vi "Cocktail.vi"() -> ()   [LabVIEW 2018]
uses:
  pathGlobal.vi
  <vilib>/Utility/config.llb/Read Key (Double).vi
  <vilib>/Utility/config.llb/Write Key (Double).vi
  <vilib>/Utility/config.llb/NI_LVConfig.lvlib
panel:
  in  "Power":bool
  out "CREDIT":dbl
  out "power":bool
  out "PROGRESS":u16(slide) scale=0.0..5.0
  out "PRICE":string
  out "STATUS":string
  out "Ingredients Panel":T1 {"JUICE" scale=0.0..2000.0; "SUGAR" scale=0.0..2000.0; "WATER" scale=0.0..2000.0; "COKE" scale=0.0..2000.0; "LIME" scale=0.0..2000.0; "WHISKY" scale=0.0..2000.0; "RUM" scale=0.0..2000.0}
  in  "0.5 €":bool
  in  "1 €":bool
  in  "2 €":bool
  in  "5 €":bool
  in  "Whisky-Cola":bool
  in  "Whisky-Sour":bool
  in  "Refill":bool
  in  "Stop":bool
  in  "Maintainance":bool
  in  "Coke":bool
  in  "Water":bool
  in  "Water-Juice":bool
  in  "Caipirinha":bool
  in  "Purchase":bool
  # "Cocktail Machine"
  # "WALLET"
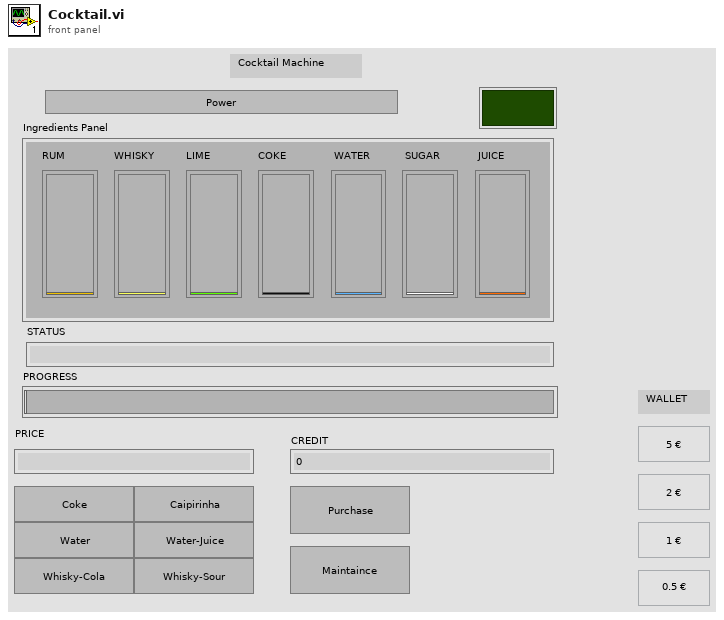
[diagram p1: front panel]
types:
  T1 = cluster{"RUM":u16, "WHISKY":u16, "LIME":u16, "COKE ":u16, " WATER":u16, " SUGAR":u16, " JUICE":u16}
  T2 = cluster{"RUM":i32, "WHISKY":i32, "LIME":i32, "COKE ":i32, " WATER":i32, " SUGAR":i32, " JUICE":i32}
  T3 = typedef "NI_LVConfig.lvlib/Config Data RefNum.ctl" = refnum<k1>
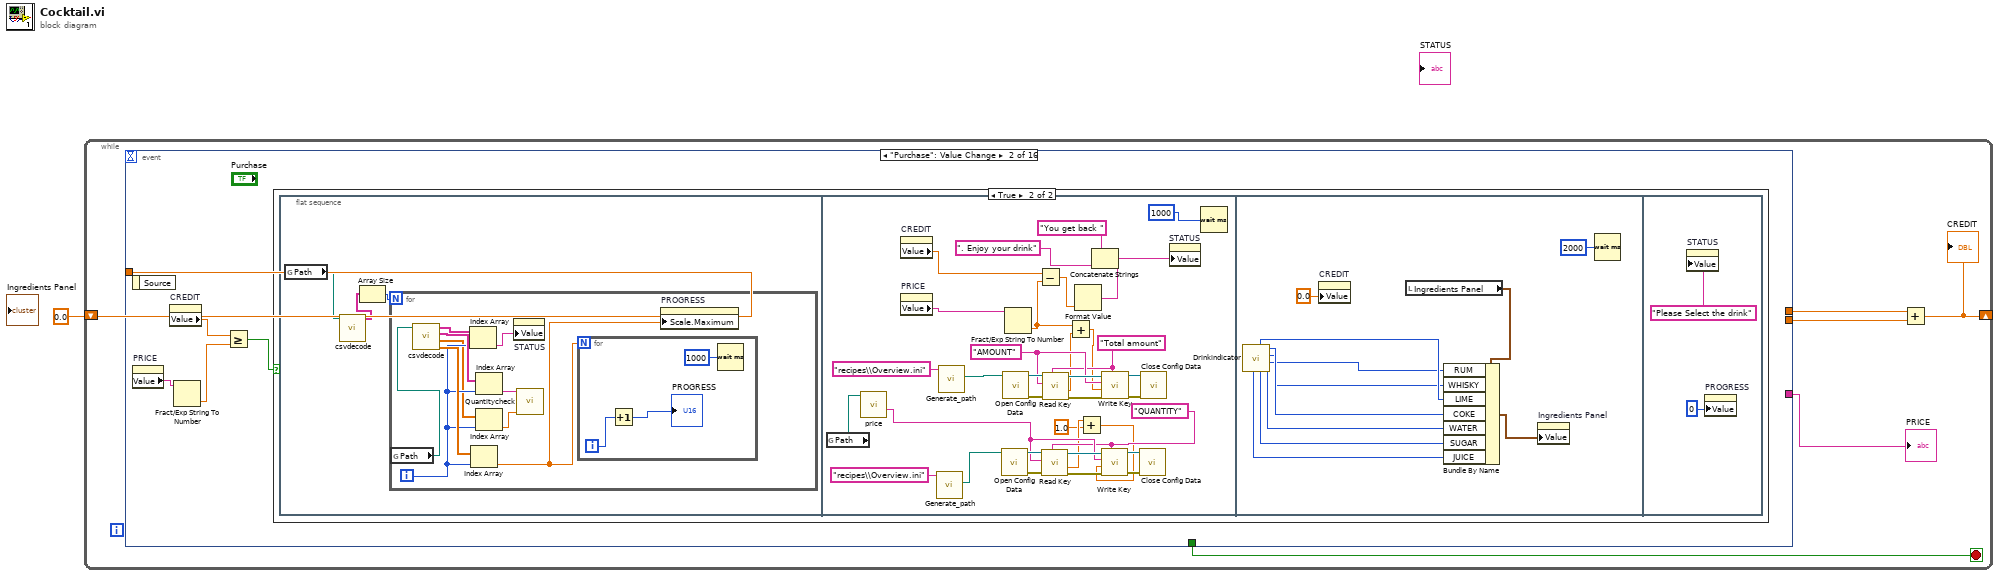
[diagram p0: block diagram]
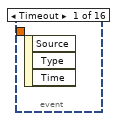
[diagram p2: hidden frame]
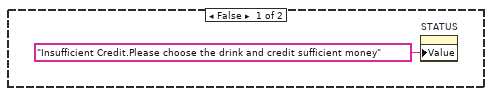
[diagram p3: hidden frame]
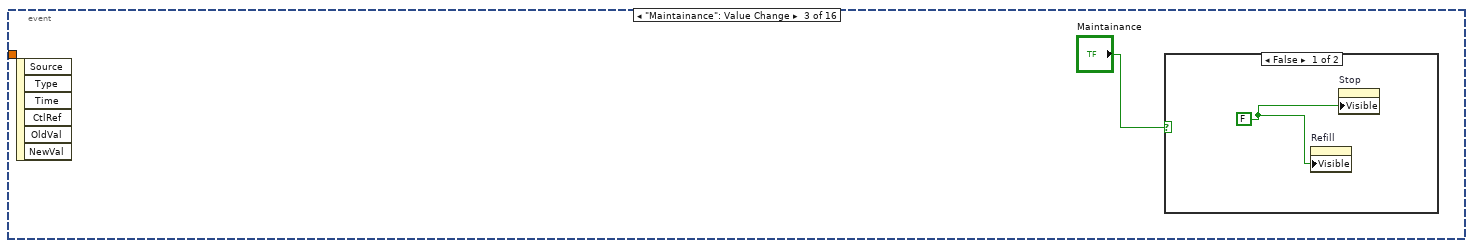
[diagram p4: hidden frame]
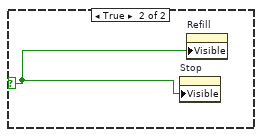
[diagram p5: hidden frame]
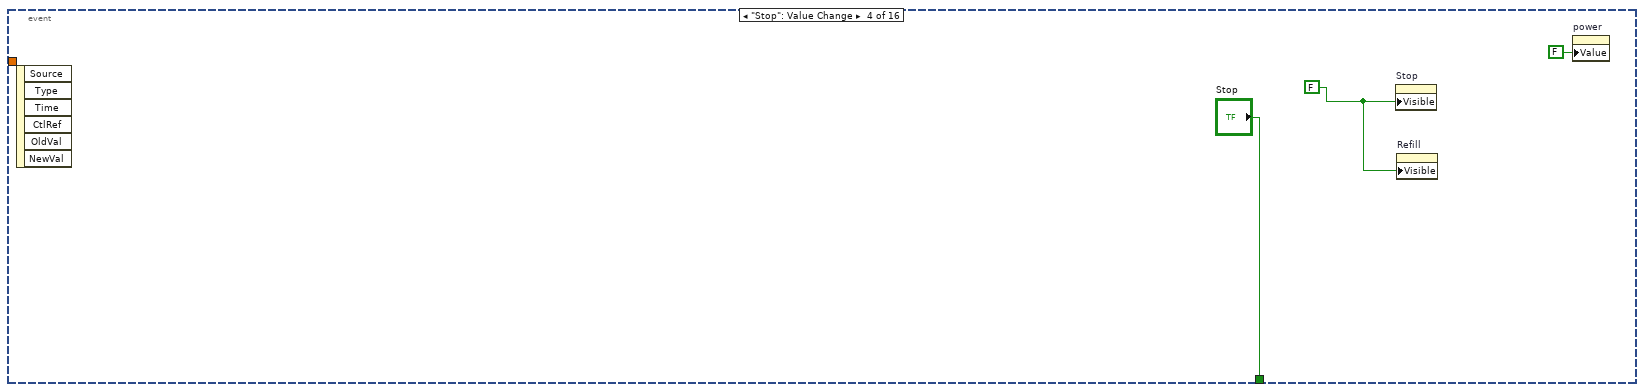
[diagram p6: hidden frame]
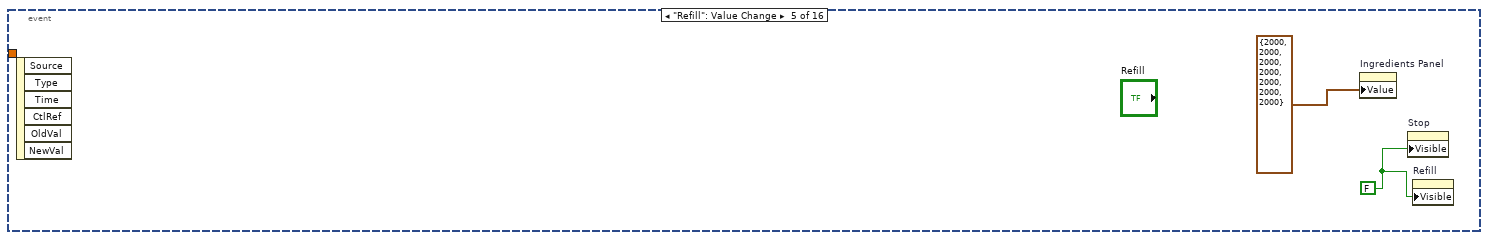
[diagram p7: hidden frame]
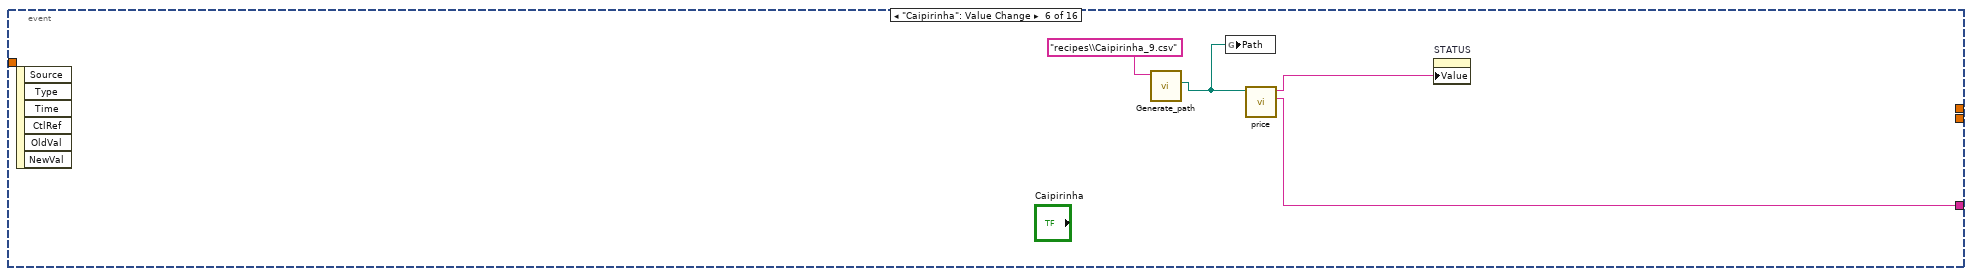
[diagram p8: hidden frame]
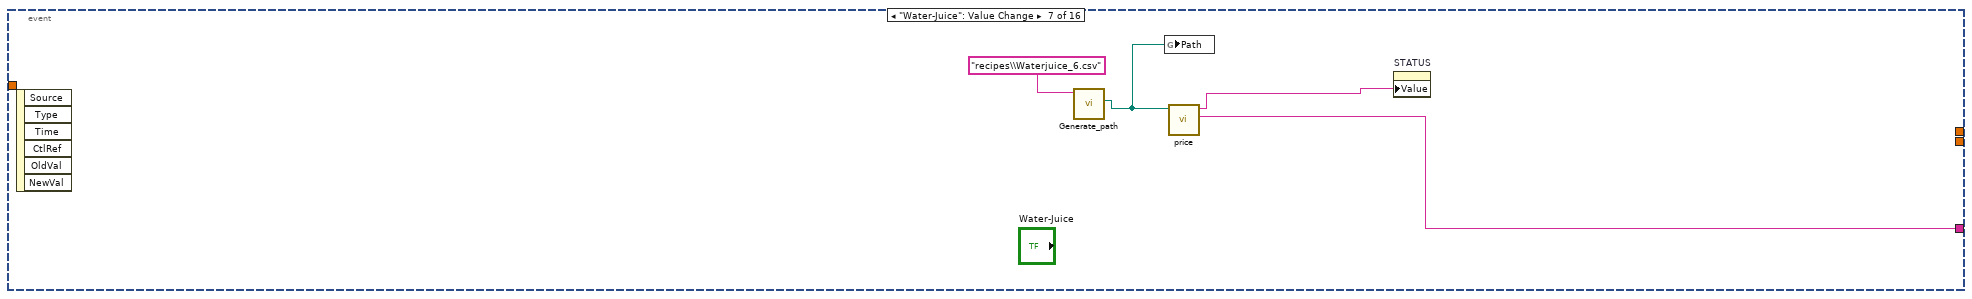
[diagram p9: hidden frame]
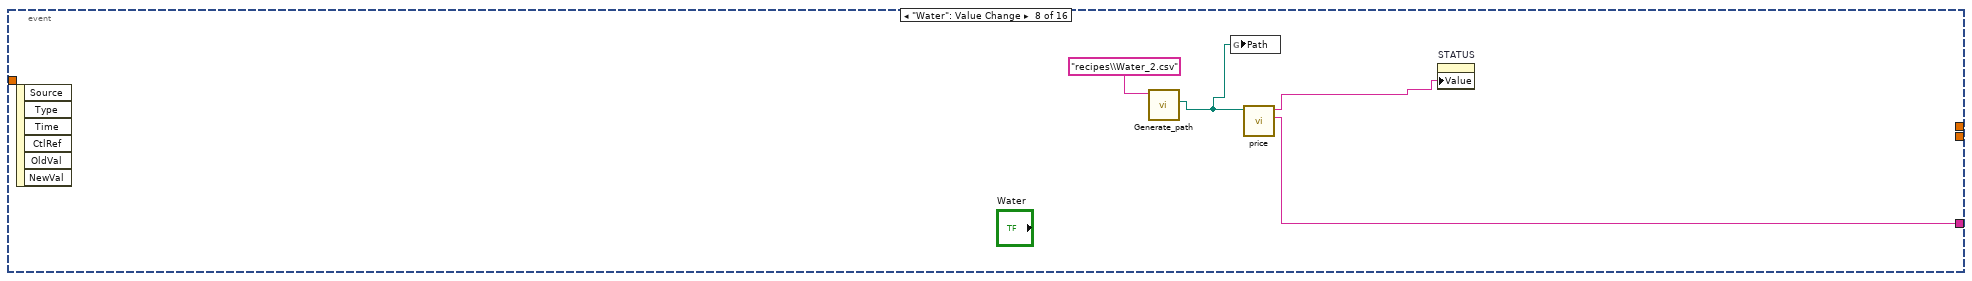
[diagram p10: hidden frame]
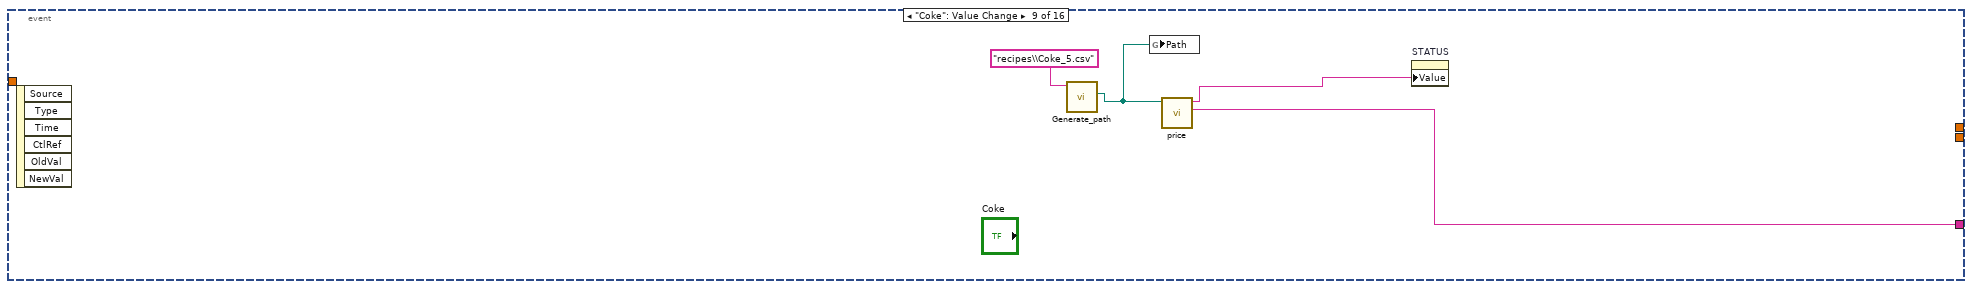
[diagram p11: hidden frame]
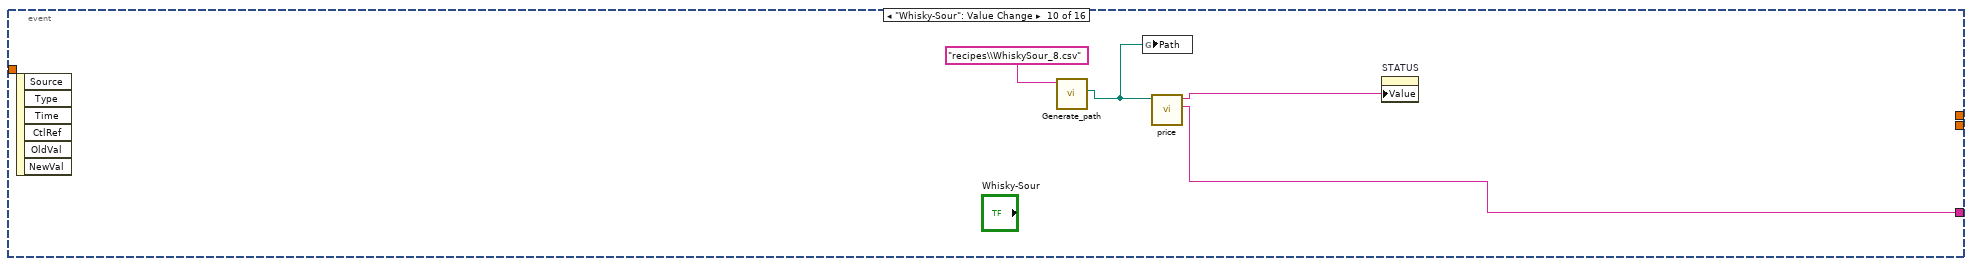
[diagram p12: hidden frame]
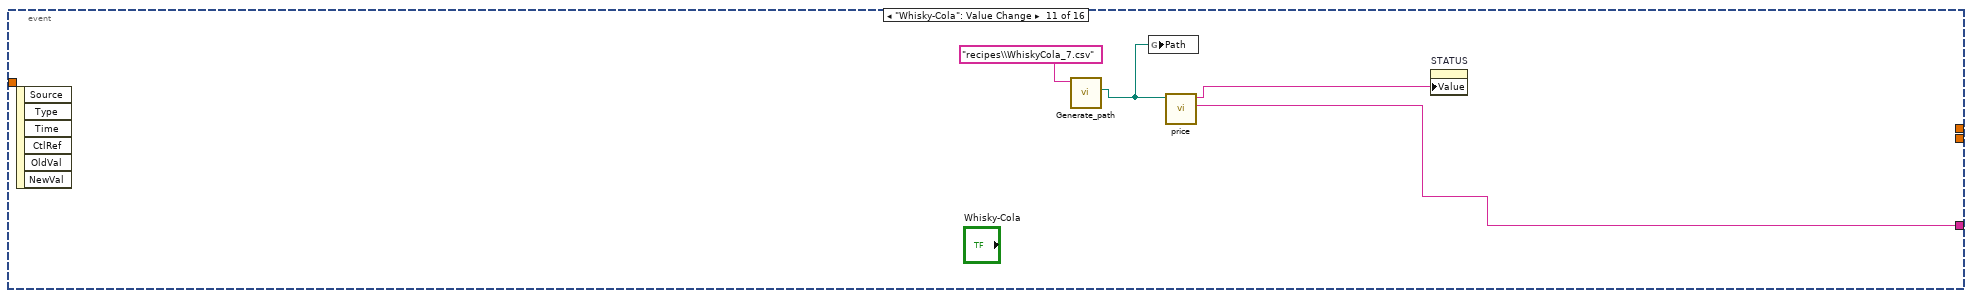
[diagram p13: hidden frame]
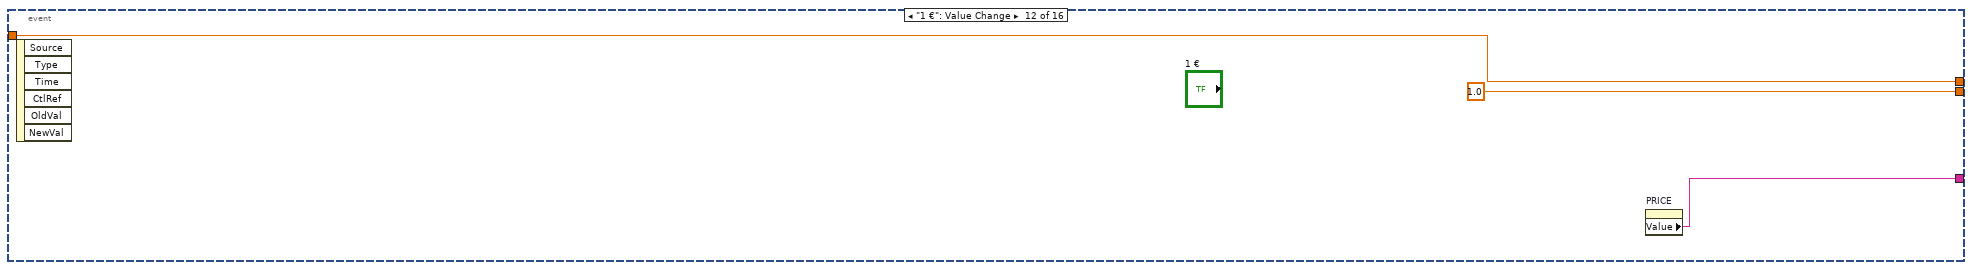
[diagram p14: hidden frame]
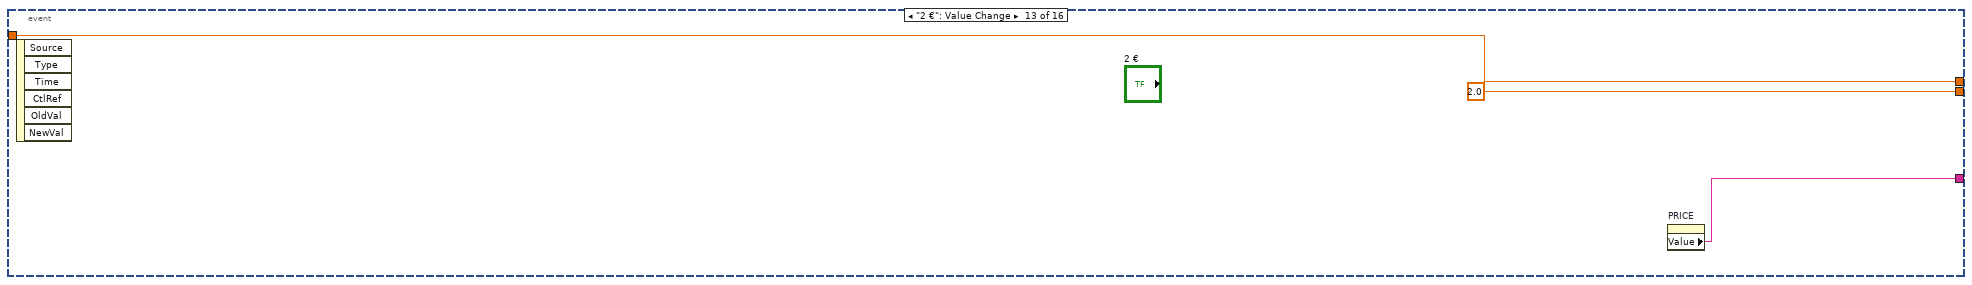
[diagram p15: hidden frame]
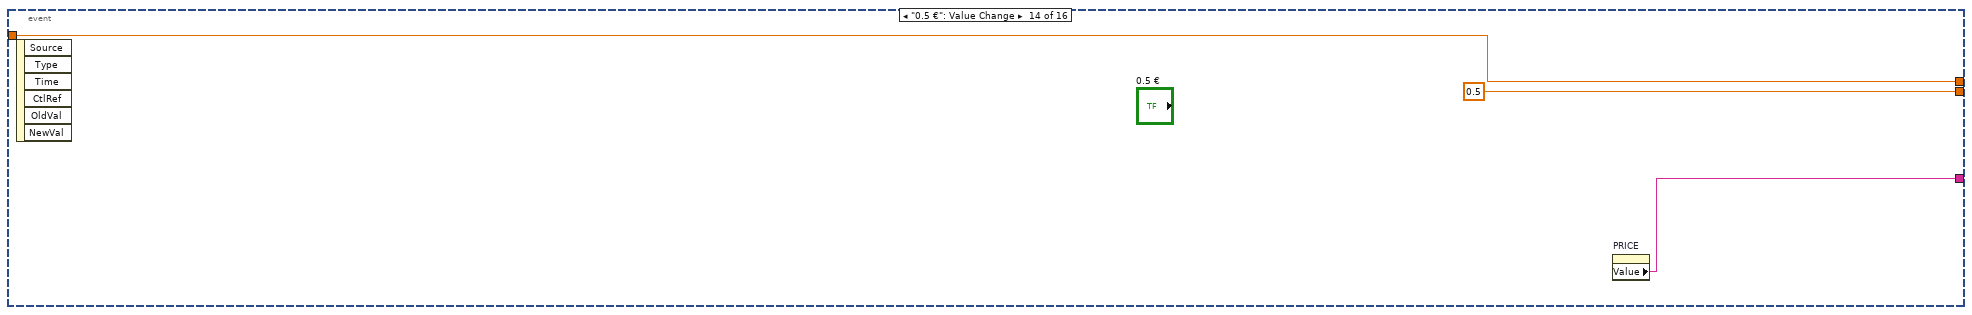
[diagram p16: hidden frame]
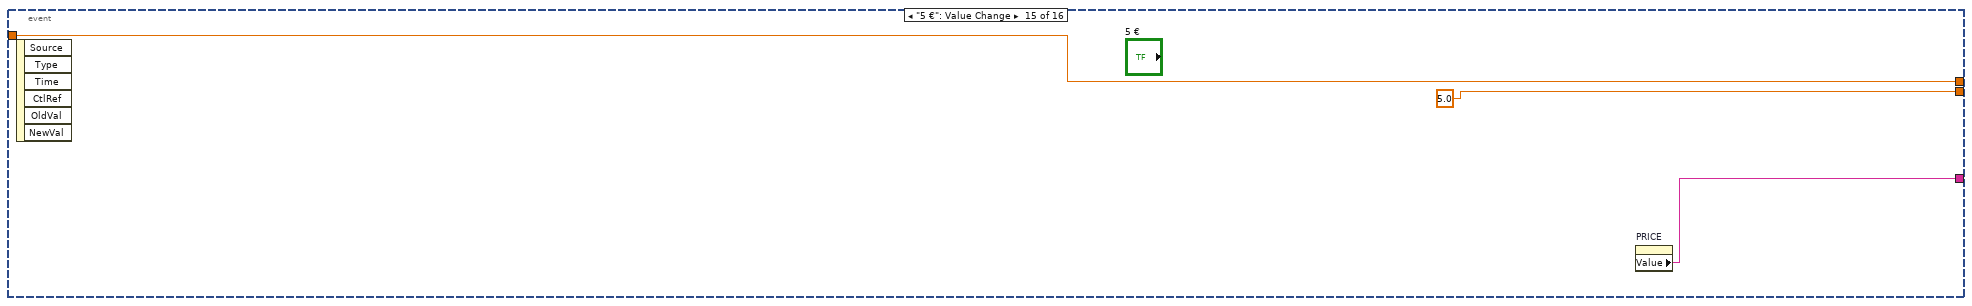
[diagram p17: hidden frame]
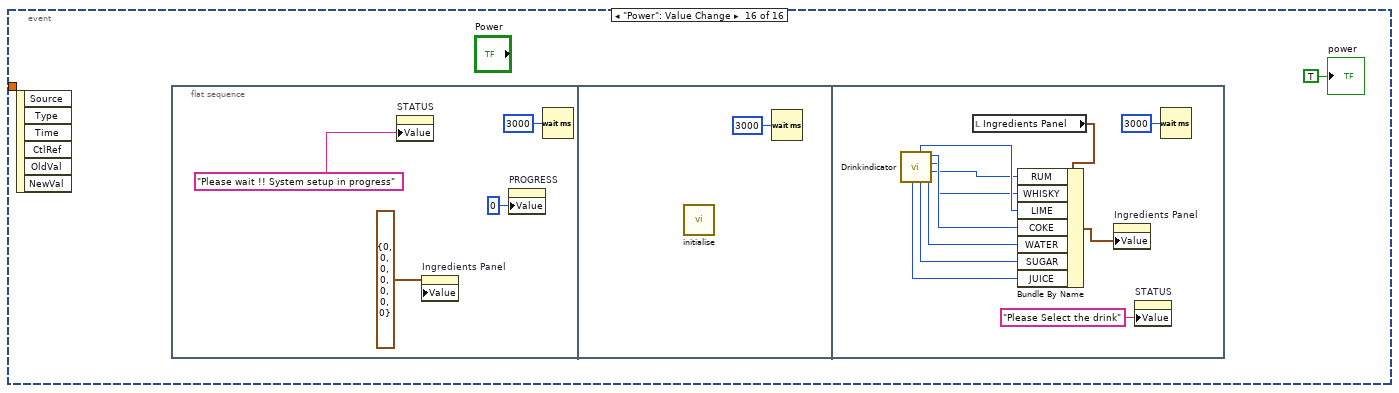
[diagram p18: hidden frame]
diagram:
  n1 = while {
    shift-right: [w6] -> _
    shift-left: 0.0 -> [w5]
    stop <- w7 stop-if-true
    n2 = event shown="[1] \"Purchase\": Value Change" {
      selector: _ -> [_ _ _ _ _ _ _ _ _ _ _ _ _ _ _ _]
      dyn-events: _ -> [_ _ _ _ _ _ _ _ _ _ _ _ _ _ _ _]
      timeout: _ -> [_ _ _ _ _ _ _ _ _ _ _ _ _ _ _ _]
      tunnel: [_ _ _ "Stop" _ _ _ _ _ _ _ _ _ _ _ _] -> w7
      tunnel: [_ _ _ _ _ _ _ _ _ _ _ w111 w114 w117 w120 _] -> w4
      tunnel: w5 -> [_ _ _ _ _ _ _ _ _ _ _ w111 w114 w117 w120 _]
      tunnel: [_ _ _ _ _ _ _ _ _ _ _ 1.0 2.0 0.5 5.0 _] -> w3
      tunnel: [_ _ _ _ _ w87 w91 w94 w98 w102 w106 w109 w112 w115 w118 _] -> w2
      event Timeout {
        n3 = event-data() -> ()  [unwired: 1 in, 3 out]
      }
      event "Purchase": Value Change {
        n4 = event-data() -> ()  [unwired: 1 in, 1 out]
        n5 = property on="PRICE" class="Str"() -> ("Value"=w11:string)  [unwired: 2 in, 2 out]
        n6 = property on="CREDIT" class="DigNum (strict)"() -> ("Value"=w10:dbl)  [unwired: 2 in, 2 out]
        n7 = Fract/Exp String To Number(string=w11) -> (number=w9:dbl)  [unwired: 3 in, 1 out]
        n8 = Greater Or Equal?(x=w10, y=w9) -> (x >= y?=w8:bool)
        n9 = case shown="True" w8 {
          frame False {
            n10 = property on="STATUS" class="Str"("Value"="Insufficient Credit.Please choose the drink and credit sufficient money" ("STATUS")) -> ()  [unwired: 2 in, 2 out]
          }
          frame True {
            n11 = flat-sequence {
              frame #0 {
                n12 = global read "pathGlobal.vi" "Path"() -> (w14:path)
                n13 = call "csvdecode.vi"("file path (dialog if empty)"=w14) -> ("Name"=w13:string[])  [unwired: 7 in, 3 out]
                n14 = Array Size(array=w13) -> (size(s)=w15:i32)
                n15 = for {
                  N: w15 -> [_]
                  i -> [w21]
                  n16 = global read "pathGlobal.vi" "Path"() -> (w16:path)
                  n17 = call "csvdecode.vi"("file path (dialog if empty)"=w16) -> ("Time"=w25:dbl[], "Quantity"=w20:dbl[], "Message"=w24:string[], "Name"=w23:string[])  [unwired: 7 in]
                  n18 = Index Array(array=w24, index=w21) -> (element=w18:string)
                  n19 = Index Array(array=w25, index=w21) -> (element=w17:dbl)
                  n20 = Index Array(array=w23, index=w21) -> (element=w22:string)
                  n21 = Index Array(array=w20, index=w21) -> (element=w19:dbl)
                  n22 = property on="STATUS" class="Str"("Value"=w18) -> ()  [unwired: 2 in, 2 out]
                  n23 = call "Quantitycheck.vi"("NUM INPUT"=w19, "key"=w22) -> ()  [unwired: 10 in]
                  n24 = for {
                    N: w17 -> [_]
                    i -> [w28]
                    n25 = Increment(x=w28) -> (x+1=→"PROGRESS":i32)
                    n26 = Wait (ms)(milliseconds to wait=u32 1000) -> ()  [unwired: 1 out]
                  }
                  n27 = property on="PROGRESS" class="Slide (strict)"("Scale.Maximum"=w17) -> ()  [unwired: 2 in, 2 out]
                }
              }
              frame #1 {
                w33 = "QUANTITY"
                w53 = "Total amount" ("section")
                w54 = "AMOUNT" ("key")
                n28 = global read "pathGlobal.vi" "Path"() -> (w43:path)
                n29 = call "price.vi"("Path"=w43) -> ("result string"=w34:string)  [unwired: 8 in, 2 out]
                n30 = property on="CREDIT" class="DigNum (strict)"() -> ("Value"=w46:dbl)  [unwired: 2 in, 2 out]
                n31 = property on="PRICE" class="Str"() -> ("Value"=w45:string)  [unwired: 2 in, 2 out]
                n32 = call "Generate_path.vi"("name or relative path"="recipes\\Overview.ini") -> ("MyFile"=w35:path)  [unwired: 10 in]
                n33 = call "Generate_path.vi"("name or relative path"="recipes\\Overview.ini") -> ("MyFile"=w47:path)  [unwired: 10 in]
                n34 = call <vilib>:"Open Config Data.vi"("configuration file path"=w35) -> ("error out"=w40:errorcluster, "refnum"=w39:T3)  [unwired: 8 in, 1 out]
                n35 = call <vilib>:"Open Config Data.vi"("configuration file path"=w47) -> ("error out"=w57:errorcluster, "refnum"=w58:T3)  [unwired: 8 in, 1 out]
                n36 = Fract/Exp String To Number(string=w45) -> (number=w49:dbl)  [unwired: 3 in, 1 out]
                n37 = Subtract(x=w46, y=w49) -> (x-y=w52:dbl)
                n38 = call-poly <vilib>:"Read Key.vi"("section"=w33, "error in (no error)"=w40, "key"=w34, "refnum"=w39) -> ("error out"=w42:errorcluster, "value"=w32:dbl, "refnum out"=w41:T3)  [unwired: 4 in, 1 out]
                n39 = call-poly <vilib>:"Read Key.vi"("section"=w53, "error in (no error)"=w57, "key"=w54, "refnum"=w58) -> ("error out"=w55:errorcluster, "value"=w51:dbl, "refnum out"=w56:T3)  [unwired: 4 in, 1 out]
                n40 = Add(x=w49, y=w51) -> (x+y=w50:dbl)
                n41 = Format Value(value (0)=w52) -> (output string=w62:string)  [unwired: 2 in]
                n42 = Add(x=w32, y=1.0 ("x")) -> (x+y=w30:dbl)
                n43 = Concatenate Strings("You get back " ("string"), w62, ". Enjoy your drink" ("string")) -> (w44:string)
                n44 = call-poly <vilib>:"Write Key.vi"("section"=w33, "error in (no error)"=w42, "value"=w30, "key"=w34, "refnum"=w41) -> ("error out"=w38:errorcluster, "refnum out"=w37:T3)  [unwired: 4 in, 1 out]
                n45 = call-poly <vilib>:"Write Key.vi"("section"=w53, "error in (no error)"=w55, "value"=w50, "key"=w54, "refnum"=w56) -> ("error out"=w59:errorcluster, "refnum out"=w60:T3)  [unwired: 4 in, 1 out]
                n46 = call <vilib>:"Close Config Data.vi"("error in (no error)"=w38, "refnum"=w37) -> ()  [unwired: 8 in, 2 out]
                n47 = call <vilib>:"Close Config Data.vi"("error in (no error)"=w59, "refnum"=w60) -> ()  [unwired: 8 in, 2 out]
                n48 = property on="STATUS" class="Str"("Value"=w44) -> ()  [unwired: 2 in, 2 out]
                n49 = Wait (ms)(milliseconds to wait=u32 1000) -> ()  [unwired: 1 out]
              }
              frame #2 {
                n50 = call "Drinkindicator.vi"() -> ("water"=w68:u32, "rum"=w69:u32, "wisky"=w70:u32, "coke"=w71:u32, "sugar"=w67:u32, "lime"=w72:u32, "juice"=w66:u32)  [unwired: 5 in]
                n51 = property on="CREDIT" class="DigNum (strict)"("Value"=0.0 ("CREDIT")) -> ()  [unwired: 2 in, 2 out]
                n52 = local read "Ingredients Panel"() -> (w73:T1)
                n53 = Bundle By Name(cluster=w73, "RUM"=w69, "WHISKY"=w70, "LIME"=w72, "COKE"=w71, "WATER"=w68, "SUGAR"=w67, "JUICE"=w66) -> (w65:T1)
                n54 = property on="Ingredients Panel" class="Clust (strict)"("Value"=w65) -> ()  [unwired: 2 in, 2 out]
                n55 = Wait (ms)(milliseconds to wait=u32 2000) -> ()  [unwired: 1 out]
              }
              frame #3 {
                n56 = property on="STATUS" class="Str"("Value"="Please Select the drink" ("STATUS")) -> ()  [unwired: 2 in, 2 out]
                n57 = property on="PROGRESS" class="Slide (strict)"("Value"=u16 0 ("PROGRESS")) -> ()  [unwired: 2 in, 2 out]
              }
            }
          }
        }
      }
      event "Maintainance": Value Change {
        n58 = event-data() -> ()  [unwired: 1 in, 6 out]
        n59 = case shown="False" "Maintainance" {
          selector: "Maintainance" -> [_ w79]
          frame False {
            w78 = FALSE
            n60 = property on="Refill" class="Bool"("Visible"=w78) -> ()  [unwired: 2 in, 2 out]
            n61 = property on="Stop" class="Bool"("Visible"=w78) -> ()  [unwired: 2 in, 2 out]
          }
          frame True {
            n62 = property on="Stop" class="Bool"("Visible"=w79) -> ()  [unwired: 2 in, 2 out]
            n63 = property on="Refill" class="Bool"("Visible"=w79) -> ()  [unwired: 2 in, 2 out]
          }
        }
      }
      event "Stop": Value Change {
        w81 = FALSE
        n64 = event-data() -> ()  [unwired: 1 in, 6 out]
        n65 = property on="Stop" class="Bool"("Visible"=w81) -> ()  [unwired: 2 in, 2 out]
        n66 = property on="Refill" class="Bool"("Visible"=w81) -> ()  [unwired: 2 in, 2 out]
        n67 = property on="power" class="Bool (strict)"("Value"=FALSE ("power")) -> ()  [unwired: 2 in, 2 out]
      }
      event "Refill": Value Change {
        w83 = FALSE
        n68 = event-data() -> ()  [unwired: 1 in, 6 out]
        n69 = property on="Ingredients Panel" class="Clust (strict)"("Value"=T2 {"RUM"=2000, "WHISKY"=2000, "LIME"=2000, "COKE "=2000, " WATER"=2000, " SUGAR"=2000, " JUICE"=2000} ("Ingredients Panel")) -> ()  [unwired: 2 in, 2 out]
        n70 = property on="Stop" class="Bool"("Visible"=w83) -> ()  [unwired: 2 in, 2 out]
        n71 = property on="Refill" class="Bool"("Visible"=w83) -> ()  [unwired: 2 in, 2 out]
      }
      event "Caipirinha": Value Change {
        n72 = event-data() -> ()  [unwired: 1 in, 6 out]
        n73 = call "Generate_path.vi"("name or relative path"="recipes\\Caipirinha_9.csv") -> ("MyFile"=w85:path)  [unwired: 10 in]
        n74 = global write "pathGlobal.vi" "Path"(w85) -> ()
        n75 = call "price.vi"("Path"=w85) -> ("match substring"=w87:string, "RESULT"=w86:string)  [unwired: 8 in, 1 out]
        n76 = property on="STATUS" class="Str"("Value"=w86) -> ()  [unwired: 2 in, 2 out]
      }
      event "Water-Juice": Value Change {
        n77 = event-data() -> ()  [unwired: 1 in, 6 out]
        n78 = call "Generate_path.vi"("name or relative path"="recipes\\Waterjuice_6.csv") -> ("MyFile"=w89:path)  [unwired: 10 in]
        n79 = global write "pathGlobal.vi" "Path"(w89) -> ()
        n80 = call "price.vi"("Path"=w89) -> ("match substring"=w91:string, "RESULT"=w90:string)  [unwired: 8 in, 1 out]
        n81 = property on="STATUS" class="Str"("Value"=w90) -> ()  [unwired: 2 in, 2 out]
      }
      event "Water": Value Change {
        n82 = event-data() -> ()  [unwired: 1 in, 6 out]
        n83 = call "Generate_path.vi"("name or relative path"="recipes\\Water_2.csv") -> ("MyFile"=w93:path)  [unwired: 10 in]
        n84 = global write "pathGlobal.vi" "Path"(w93) -> ()
        n85 = call "price.vi"("Path"=w93) -> ("match substring"=w94:string, "RESULT"=w95:string)  [unwired: 8 in, 1 out]
        n86 = property on="STATUS" class="Str"("Value"=w95) -> ()  [unwired: 2 in, 2 out]
      }
      event "Coke": Value Change {
        n87 = event-data() -> ()  [unwired: 1 in, 6 out]
        n88 = call "Generate_path.vi"("name or relative path"="recipes\\Coke_5.csv") -> ("MyFile"=w97:path)  [unwired: 10 in]
        n89 = global write "pathGlobal.vi" "Path"(w97) -> ()
        n90 = call "price.vi"("Path"=w97) -> ("match substring"=w98:string, "RESULT"=w99:string)  [unwired: 8 in, 1 out]
        n91 = property on="STATUS" class="Str"("Value"=w99) -> ()  [unwired: 2 in, 2 out]
      }
      event "Whisky-Sour": Value Change {
        n92 = event-data() -> ()  [unwired: 1 in, 6 out]
        n93 = call "Generate_path.vi"("name or relative path"="recipes\\WhiskySour_8.csv") -> ("MyFile"=w101:path)  [unwired: 10 in]
        n94 = global write "pathGlobal.vi" "Path"(w101) -> ()
        n95 = call "price.vi"("Path"=w101) -> ("match substring"=w102:string, "RESULT"=w103:string)  [unwired: 8 in, 1 out]
        n96 = property on="STATUS" class="Str"("Value"=w103) -> ()  [unwired: 2 in, 2 out]
      }
      event "Whisky-Cola": Value Change {
        n97 = event-data() -> ()  [unwired: 1 in, 6 out]
        n98 = call "Generate_path.vi"("name or relative path"="recipes\\WhiskyCola_7.csv") -> ("MyFile"=w105:path)  [unwired: 10 in]
        n99 = global write "pathGlobal.vi" "Path"(w105) -> ()
        n100 = call "price.vi"("Path"=w105) -> ("match substring"=w106:string, "RESULT"=w107:string)  [unwired: 8 in, 1 out]
        n101 = property on="STATUS" class="Str"("Value"=w107) -> ()  [unwired: 2 in, 2 out]
      }
      event "1 €": Value Change {
        n102 = event-data() -> ()  [unwired: 1 in, 6 out]
        n103 = property on="PRICE" class="Str"() -> ("Value"=w109:string)  [unwired: 2 in, 2 out]
      }
      event "2 €": Value Change {
        n104 = event-data() -> ()  [unwired: 1 in, 6 out]
        n105 = property on="PRICE" class="Str"() -> ("Value"=w112:string)  [unwired: 2 in, 2 out]
      }
      event "0.5 €": Value Change {
        n106 = event-data() -> ()  [unwired: 1 in, 6 out]
        n107 = property on="PRICE" class="Str"() -> ("Value"=w115:string)  [unwired: 2 in, 2 out]
      }
      event "5 €": Value Change {
        n108 = event-data() -> ()  [unwired: 1 in, 6 out]
        n109 = property on="PRICE" class="Str"() -> ("Value"=w118:string)  [unwired: 2 in, 2 out]
      }
      event "Power": Value Change {
        n110 = event-data() -> ()  [unwired: 1 in, 6 out]
        n111 = flat-sequence {
          frame #0 {
            n112 = property on="STATUS" class="Str"("Value"="Please wait !! System setup in progress") -> ()  [unwired: 2 in, 2 out]
            n113 = property on="Ingredients Panel" class="Clust (strict)"("Value"=T1 {"RUM"=0, "WHISKY"=0, "LIME"=0, "COKE "=0, " WATER"=0, " SUGAR"=0, " JUICE"=0} ("Ingredients Panel")) -> ()  [unwired: 2 in, 2 out]
            n114 = property on="PROGRESS" class="Slide (strict)"("Value"=u16 0 ("PROGRESS")) -> ()  [unwired: 2 in, 2 out]
            n115 = Wait (ms)(milliseconds to wait=u32 3000) -> ()  [unwired: 1 out]
          }
          frame #1 {
            n116 = call "initialise.vi"() -> ()  [unwired: 12 in]
            n117 = Wait (ms)(milliseconds to wait=u32 3000) -> ()  [unwired: 1 out]
          }
          frame #2 {
            n118 = call "Drinkindicator.vi"() -> ("water"=w132:u32, "rum"=w133:u32, "wisky"=w134:u32, "coke"=w135:u32, "sugar"=w131:u32, "lime"=w136:u32, "juice"=w130:u32)  [unwired: 5 in]
            n119 = local read "Ingredients Panel"() -> (w137:T1)
            n120 = Bundle By Name(cluster=w137, "RUM"=w133, "WHISKY"=w134, "LIME"=w136, "COKE"=w135, "WATER"=w132, "SUGAR"=w131, "JUICE"=w130) -> (w127:T1)
            n121 = property on="Ingredients Panel" class="Clust (strict)"("Value"=w127) -> ()  [unwired: 2 in, 2 out]
            n122 = property on="STATUS" class="Str"("Value"="Please Select the drink" ("STATUS")) -> ()  [unwired: 2 in, 2 out]
            n123 = Wait (ms)(milliseconds to wait=u32 3000) -> ()  [unwired: 1 out]
          }
        }
        "power" <- TRUE ("power")
      }
    }
    "PRICE" <- w2
    n124 = Add(x=w4, y=w3) -> (x+y=w6:dbl)
    "CREDIT" <- w6
  }
